vi "Update Force Bytes.vi"(8 "error in (no error)":errorcluster, 10 "FATypes":T1, 11 "Model in":refnum<class "Model.lvclass">) -> (0 "error out":errorcluster, 3 "Model out":refnum<class "Model.lvclass">)   [LabVIEW 2016, in "Model.lvclass"]
uses:
  Model.lvclass
  Common_RT_FAILC/DataTypes/FATypes.ctl
  Model.lvclass/Model.ctl
  Modbus/DesktopModbus/DesktopModbus.lvclass/DesktopModbus.ctl
  Modbus/DesktopModbus/DesktopModbus.lvclass
  Common_RT_FAILC/RTFAILC.lvlib
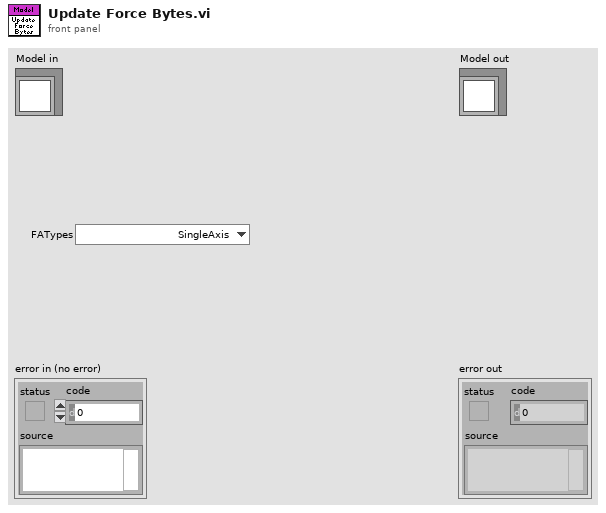
[diagram p1: front panel]
types:
  T1 = typedef "RTFAILC.lvlib/FATypes.ctl" = enum16{"SingleAxis", "LateralDualAxis", "CrossLateralDualAxis"}
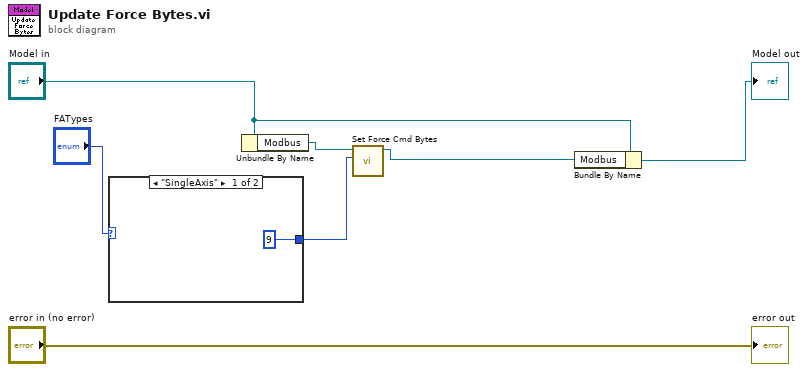
[diagram p0: block diagram]
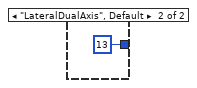
[diagram p2: hidden frame]
diagram:
  n1 = case shown="\"SingleAxis\"" "FATypes" {
    tunnel: [9 13] -> w1
    frame "SingleAxis" {
    }
    frame "LateralDualAxis", Default {
    }
  }
  n2 = Unbundle By Name("Model in") -> ("Modbus"=w7:refnum<class "DesktopModbus.lvclass">)
  n3 = call "Set Force Cmd Bytes.vi"("ForceCmdBytes"=w1, "DesktopModbus in"=w7) -> ("DesktopModbus out"=w6:refnum<class "DesktopModbus.lvclass">)  [unwired: 9 in]
  n4 = Bundle By Name(cluster="Model in", "Modbus"=w6) -> (→"Model out":refnum<class "Model.lvclass">)
  "error out" <- "error in (no error)"
